vi "Intensity Graph to XY Graph (Vertical) (by val).vi"(8 "error in (no error)":errorcluster, 10 "2D Data":dbl[][](array[numeric]), 11 "graph_utilities in":refnum<class "graph_utilities.lvclass">) -> (0 "error out":errorcluster, 2 "XY-data":cluster{"X-array":dbl[], "Y-array":dbl[]}[](array[cluster]), 3 "graph_utilities out":refnum<class "graph_utilities.lvclass">)   [LabVIEW 2019, in "graph_utilities.lvclass"]
doc: "Converts an Intensity Graph into a sequence of plots on a XY Graph.\n\nThe x-axis of the XY Graph will be equal to the y-axis of the Intensity Graph."
uses:
  graph_utilities.lvclass
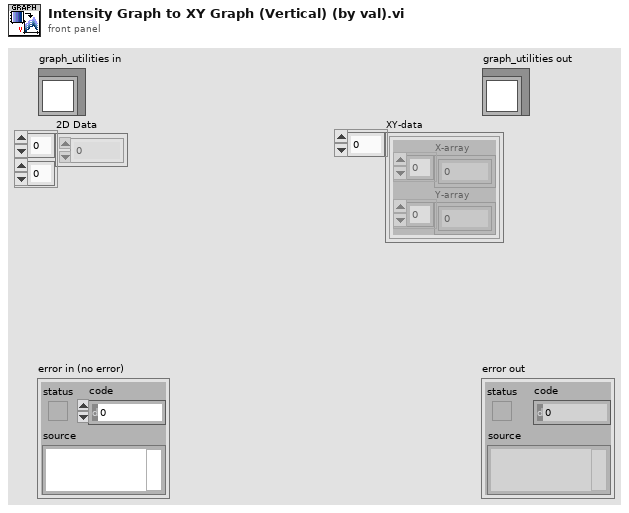
[diagram p1: front panel]
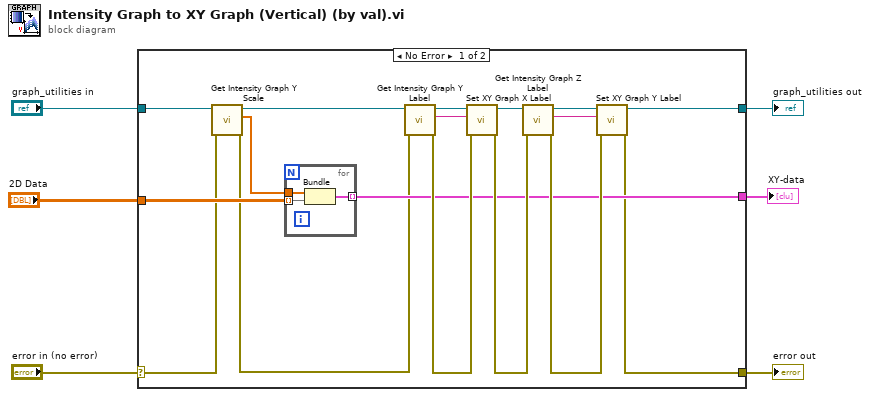
[diagram p0: block diagram]
diagram:
  n1 = case shown="No Error" "error in (no error)" {
    selector: "error in (no error)" -> [w7 w28]
    tunnel: [w9 w28] -> w5
    tunnel: [w13 w27] -> w3
    tunnel: "graph_utilities in" -> [w11 w27]
    tunnel: "2D Data" -> [w12 _]
    tunnel: [w10 _] -> w1
    frame No Error {
      n2 = call "Get Intensity Graph Y Scale.vi"("error in (no error)"=w7, "graph_utilities in"=w11) -> ("error out"=w8:errorcluster, "Y Scale"=w23:dbl[], "graph_utilities out"=w22:refnum<class "graph_utilities.lvclass">)  [unwired: 6 in, 1 out]
      n3 = for {
        tunnel: w12 -> [w25] mode=indexing
        tunnel: w23 -> [w26]
        tunnel: [w24] -> w10 mode=indexing
        n4 = Bundle("Y Scale"=w26, "2D Data"=w25) -> (w24:cluster{"Y Scale":dbl[], "2D Data":dbl[]})  [unwired: 1 in]
      }
      n5 = call "Get Intensity Graph Y Label.vi"("error in (no error)"=w8, "graph_utilities in"=w22) -> ("error out"=w15:errorcluster, "Y Label"=w21:string, "graph_utilities out"=w16:refnum<class "graph_utilities.lvclass">)  [unwired: 7 in]
      n6 = call "Set XY Graph X Label.vi"("error in (no error)"=w15, "X Label"=w21, "graph_utilities in"=w16) -> ("error out"=w17:errorcluster, "graph_utilities out"=w18:refnum<class "graph_utilities.lvclass">)  [unwired: 7 in]
      n7 = call "Get Intensity Graph Z Label.vi"("error in (no error)"=w17, "graph_utilities in"=w18) -> ("error out"=w14:errorcluster, "Z Label"=w20:string, "graph_utilities out"=w19:refnum<class "graph_utilities.lvclass">)  [unwired: 7 in]
      n8 = call "Set XY Graph Y Label.vi"("error in (no error)"=w14, "Y Label"=w20, "graph_utilities in"=w19) -> ("error out"=w9:errorcluster, "graph_utilities out"=w13:refnum<class "graph_utilities.lvclass">)  [unwired: 7 in]
    }
    frame Error {
    }
  }
  "error out" <- w5
  "graph_utilities out" <- w3
  "XY-data" <- w1
